vi "GetSize.vi"(8 "error in (no error)":errorcluster, 11 "reference in":refnum<class "mmWave data.lvclass">) -> (0 "error out":errorcluster, 1 "Size (Bytes)":dbl, 2 "Size":i32, 3 "reference out":refnum<class "mmWave data.lvclass">)   [LabVIEW 2019, in "mmWave data.lvclass"]
doc: "Returns number of samples of IQ waveform"
uses:
  mmWave data.lvclass
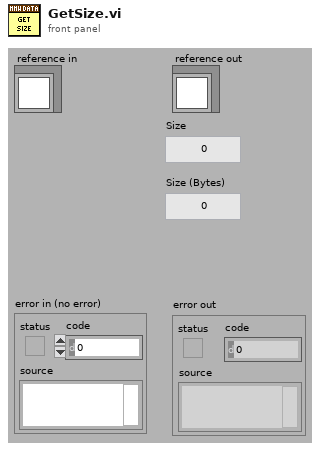
[diagram p1: front panel]
types:
  T1 = typedef "mmWave data.lvclass/ObjectAttributes.ctl" = cluster{"MyAttribute":dbl, "size":i32}
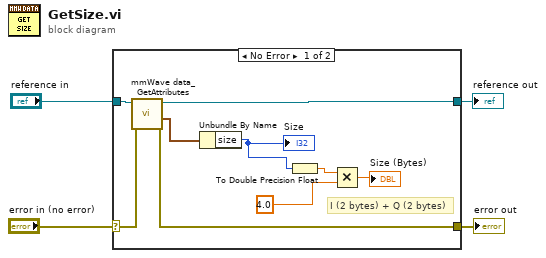
[diagram p0: block diagram]
diagram:
  n1 = case shown="No Error" "error in (no error)" {
    selector: "error in (no error)" -> [w13 w15]
    tunnel: [w12 w15] -> w3
    tunnel: [w11 w14] -> w1
    tunnel: "reference in" -> [w9 w14]
    frame No Error {
      # "I (2 bytes) + Q (2 bytes)"
      n2 = call "mmWave data_GetAttributes.vi"("error in (no error)"=w13, "reference in"=w9) -> ("error out"=w12:errorcluster, "attributes"=w10:T1, "reference out"=w11:refnum<class "mmWave data.lvclass">)  [unwired: 6 in, 1 out]
      n3 = Unbundle By Name(w10) -> ("size"=w7:i32)
      "Size" <- w7
      n4 = To Double Precision Float(number=w7) -> (double precision float=w6:dbl)
      n5 = Multiply(x=w6, y=4.0) -> (x*y=→"Size (Bytes)":dbl)
    }
    frame Error {
    }
  }
  "error out" <- w3
  "reference out" <- w1
